vi "Automate_de_production.vi"(1 "OK Button 2":bool, 2 "Cancel Button 2":bool, 3 "?":bool, 4 "Cancel Button":bool, 5 "OK Button":bool, 6 "Radio Buttons":enum32{"Radio Selection 1", "Radio Selection 2"}(radio), 7 "StartB":bool) -> (0 "cannettes produites":dbl)   [LabVIEW 2023]
uses:
  Control 1.ctl
  Control 5.ctl
  <vilib>/numeric/Random Number (Range) U64.vi
  <vilib>/numeric/sub_Random U32.vi
panel:
  out "Produits defectueux":dbl
  out "Produits Finis":dbl
  out "Nb cycles":dbl
  in  "OK Button 3":bool
  out "MP3 2":bool
  out "Valeur PH":dbl
  out "Boolean":bool
  in  "Seuil PH":dbl(slide) scale=0.0..14.0
  out "Tab Control":T1(tab)
  out "MP3":bool
  out "Tank":cluster{dbl, dbl}(slide)={0.0, 10.0} scale=0.0..10.0
  # "DO u want gaz ?"
  # "DO u want sugar ?"
  # "Production finie"
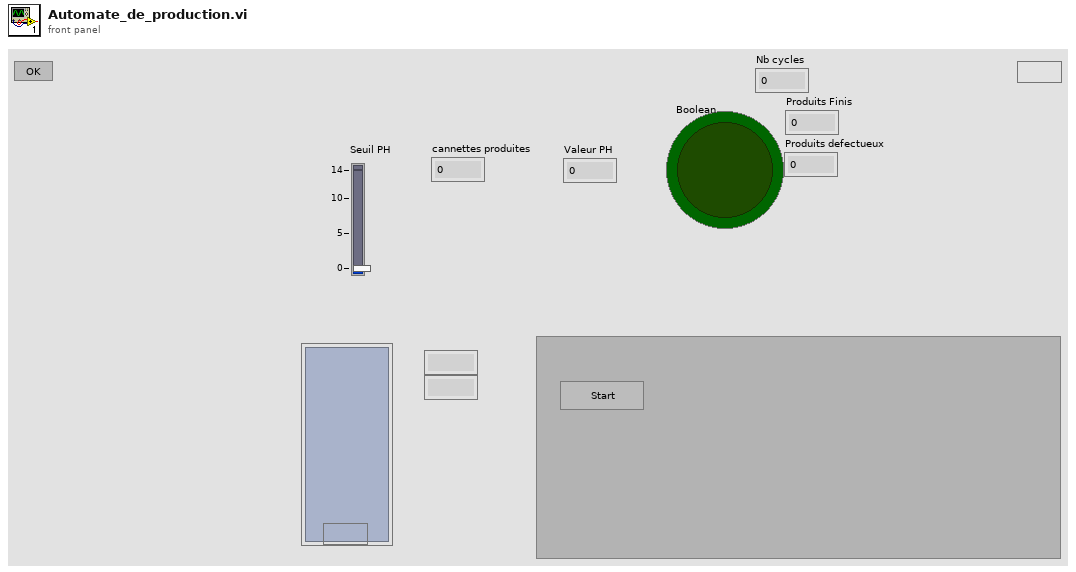
[diagram p1: front panel]
types:
  T1 = enum32{"Start", "Type", "preparer", "GazS", "GazF", "Sugar", "Finish"}
  T2 = typedef "Control 1.ctl" = enum32{"Start", "Page 1", "Page 2", "Page 3", "Page 4", "Sugar", "Finish"}
  T3 = typedef "Control 5.ctl" = enum32{"Start", "Page 1", "Page 2", "Page 3", "Page4"}
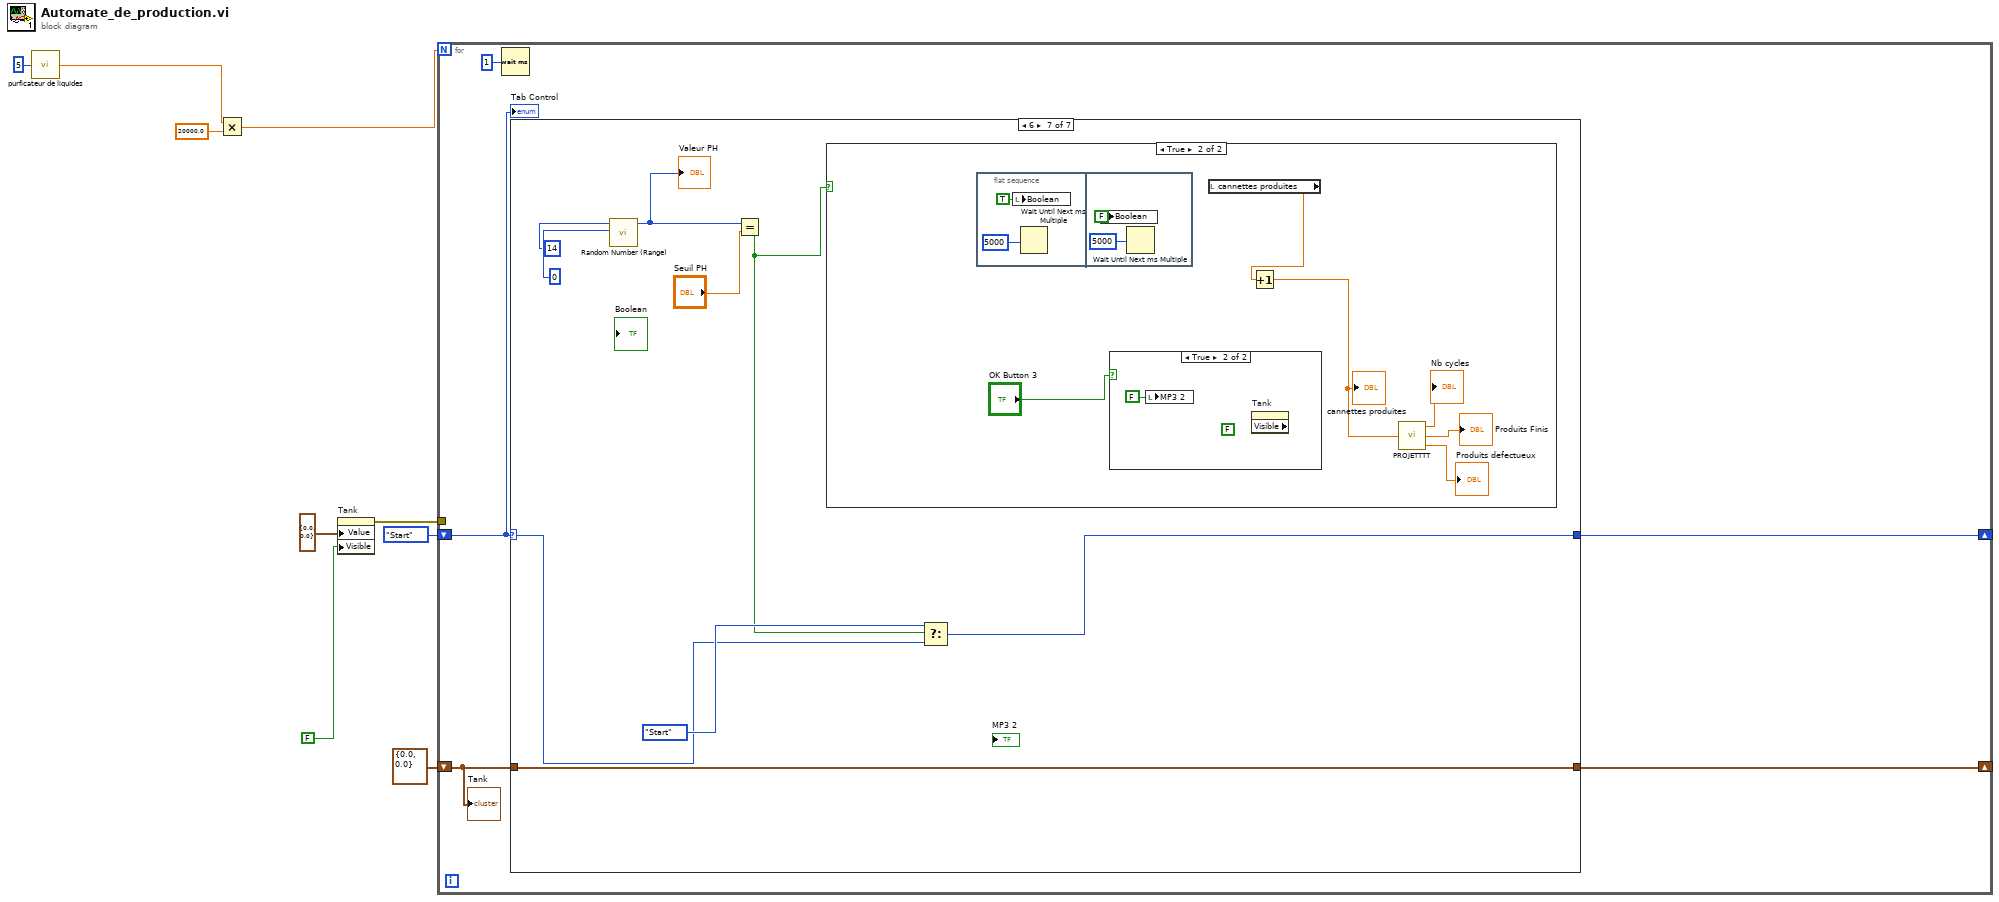
[diagram p0: block diagram]
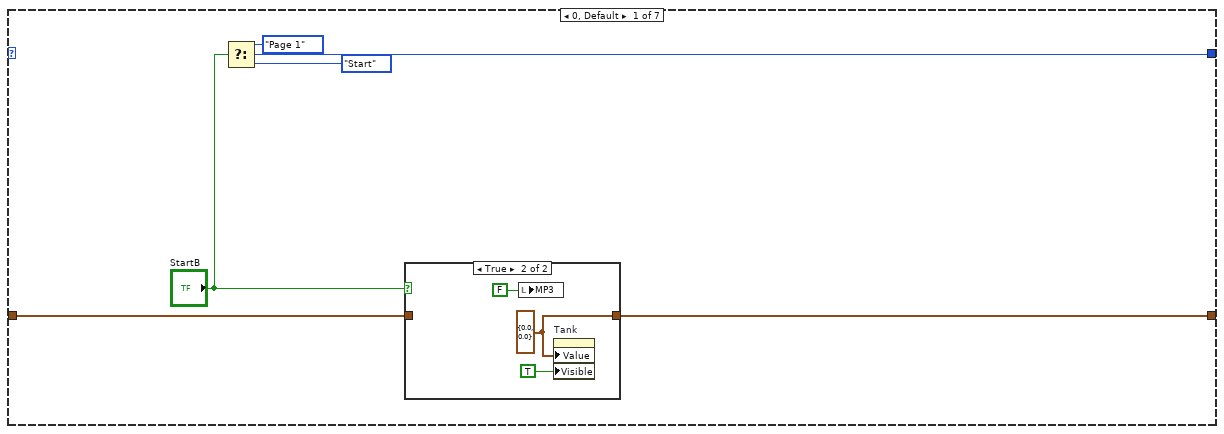
[diagram p2: hidden frame]
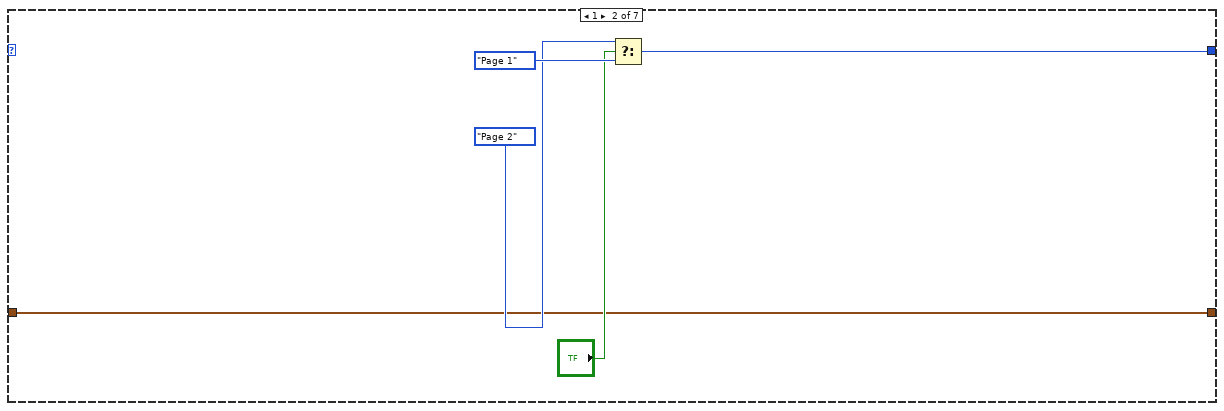
[diagram p4: hidden frame]
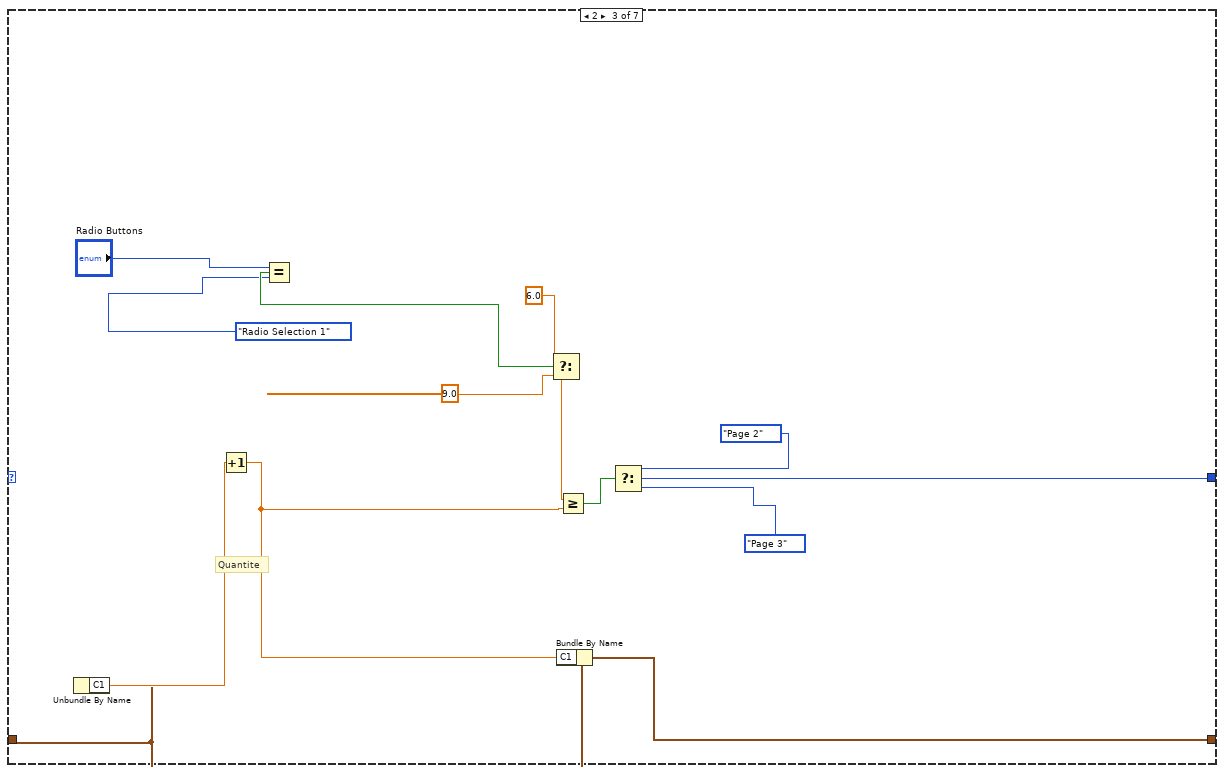
[diagram p5: hidden frame]
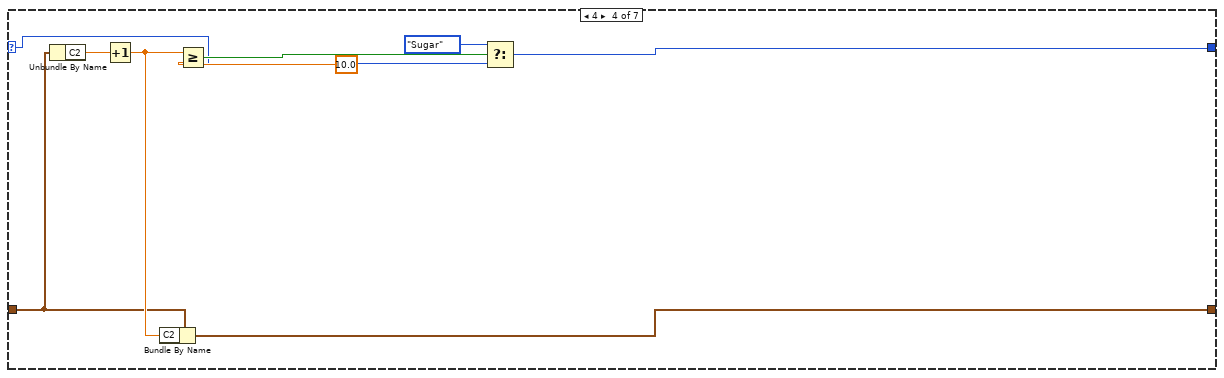
[diagram p6: hidden frame]
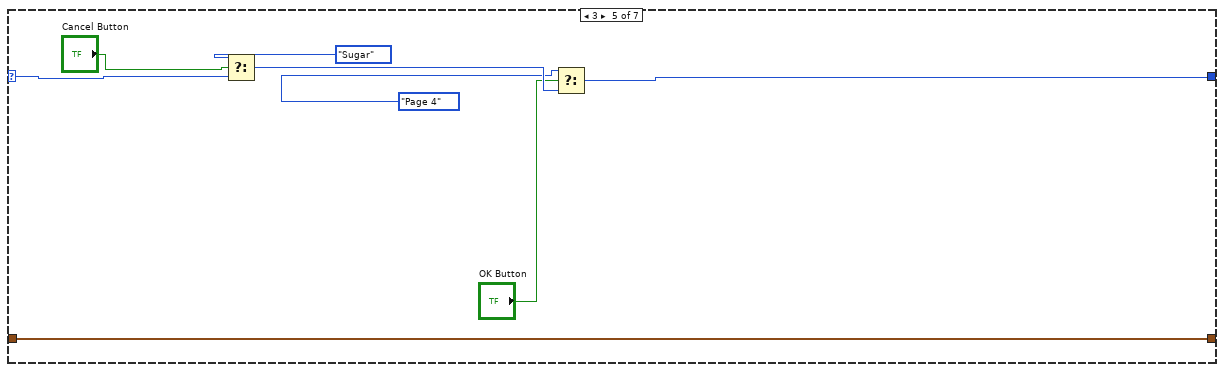
[diagram p7: hidden frame]
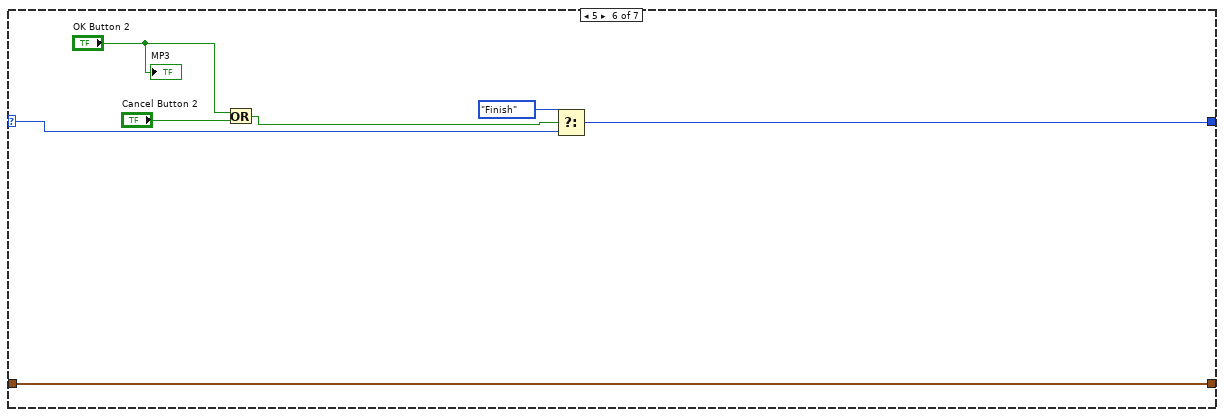
[diagram p8: hidden frame]
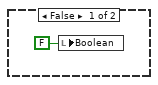
[diagram p9: hidden frame]
diagram:
  n1 = call "purficateur de liquides.vi"("Nb de litres recus"=5) -> ("nb de litres purifies"=w2:dbl)
  n2 = Multiply(x=w2, y=20000.0) -> (x*y=w3:dbl)
  n3 = property on="Tank" class="Slide (strict)"("Value"=cluster{dbl, dbl} {0.0, 0.0} ("Tank"), "Visible"=FALSE) -> (error out=w6:errorcluster)  [unwired: 2 in, 1 out]
  n4 = for {
    N: w3 -> [_]
    shift-right: [w14] -> _
    shift-left: cluster{"C1":dbl, "C2":dbl} {"C1"=0.0, "C2"=0.0} ("Tank") -> [w11]
    shift-right: [w12] -> _
    shift-left: Control_1."Start" ("Tab Control") -> [w13]
    tunnel: w6 -> [_]
    n5 = Wait (ms)(milliseconds to wait=u32 1 ("millisecond timer value")) -> ()  [unwired: 1 out]
    n6 = case shown="6" w13 {
      selector: w13 -> [_ _ _ w46 w59 w65 w74]
      tunnel: [w17 w26 w32 w44 w56 w62 w73] -> w12
      tunnel: w11 -> [w16 w25 w37 w48 w53 w67 w76]
      tunnel: [w15 w25 w36 w47 w53 w67 w76] -> w14
      frame 0, Default {
        n7 = Select(t=Control_5."Page 1" ("Tab Control"), s="StartB", f=Control_5."Start" ("Tab Control")) -> (s? t:f=w17:T3)
        n8 = case shown="True" "StartB" {
          tunnel: [w21 w22] -> w15
          tunnel: w16 -> [w21 _]
          frame False {
          }
          frame True {
            w22 = cluster{dbl, dbl} {0.0, 0.0} ("Tank")
            n9 = local write "MP3"(FALSE ("MP3")) -> ()
            n10 = property on="Tank" class="Slide (strict)"("Value"=w22, "Visible"=TRUE) -> ()  [unwired: 2 in, 2 out]
          }
        }
      }
      frame 1 {
        n11 = Select(t=Control_5."Page 2" ("Tab Control"), s="?", f=Control_5."Page 1" ("Tab Control")) -> (s? t:f=w26:T3)
      }
      frame 2 {
        # "Quantite"
        n12 = Unbundle By Name(w37) -> ("C1"=w38:dbl)
        n13 = Increment(x=w38) -> (x+1=w31:dbl)
        n14 = Equal?(x="Radio Buttons", y=enum32{"Radio Selection 1", "Radio Selection 2"}."Radio Selection 1" ("x")) -> (x = y?=w41:bool)
        n15 = Select(t=6.0, s=w41, f=9.0) -> (s? t:f=w30:dbl)
        n16 = Bundle By Name(cluster=w37, "C1"=w31) -> (w36:cluster{"C1":dbl, "C2":dbl})
        n17 = Greater Or Equal?(x=w30, y=w31) -> (x >= y?=w33:bool)
        n18 = Select(t=Control_5."Page 2" ("Tab Control"), s=w33, f=Control_5."Page 3" ("Tab Control")) -> (s? t:f=w32:T3)
      }
      frame 4 {
        n19 = Unbundle By Name(w48) -> ("C2"=w52:dbl)
        n20 = Increment(x=w52) -> (x+1=w51:dbl)
        n21 = Bundle By Name(cluster=w48, "C2"=w51) -> (w47:cluster{"C1":dbl, "C2":dbl})
        n22 = Greater Or Equal?(x=w51, y=10.0) -> (x >= y?=w50:bool)
        n23 = Select(t=Control_1."Sugar" ("Tab Control"), s=w50, f=w46) -> (s? t:f=w44:u32)
      }
      frame 3 {
        n24 = Select(t=Control_1."Sugar" ("Tab Control"), s="Cancel Button", f=w59) -> (s? t:f=w58:u32)
        n25 = Select(t=Control_1."Page 4" ("Tab Control"), s="OK Button", f=w58) -> (s? t:f=w56:u32)
      }
      frame 5 {
        n26 = Or(x="OK Button 2", y="Cancel Button 2") -> (x .or. y?=w64:bool)
        n27 = Select(t=Control_1."Finish" ("Tab Control"), s=w64, f=w65) -> (s? t:f=w62:u32)
        "MP3" <- "OK Button 2"
      }
      frame 6 {
        n28 = call-poly <vilib>:"Random Number (Range).vi"("lower bound (0)"=u64 0, "upper bound (100)"=u64 14) -> ("number"=w72:u64)  [unwired: 9 in]
        "Valeur PH" <- w72
        n29 = Equal?(x=w72, y="Seuil PH") -> (x = y?=w68:bool)
        n30 = case shown="True" w68 {
          frame False {
            n31 = local write "Boolean"(FALSE ("Boolean")) -> ()
          }
          frame True {
            n32 = flat-sequence {
              frame #0 {
                n33 = local write "Boolean"(TRUE ("Boolean")) -> ()
                n34 = Wait Until Next ms Multiple(millisecond multiple=u32 5000 ("millisecond timer value")) -> ()  [unwired: 1 out]
              }
              frame #1 {
                n35 = local write "Boolean"(FALSE ("Boolean")) -> ()
                n36 = Wait Until Next ms Multiple(millisecond multiple=u32 5000 ("millisecond timer value")) -> ()  [unwired: 1 out]
              }
            }
            n37 = case shown="True" "OK Button 3" {
              frame False {
              }
              frame True {
                (unwired) FALSE ("Visible")
                n38 = local write "MP3 2"(FALSE ("MP3")) -> ()
                n39 = property on="Tank" class="Slide (strict)" props=["Visible"]() -> ()  [unwired: 2 in, 3 out]
              }
            }
            n40 = local read "cannettes produites"() -> (w83:dbl)
            n41 = Increment(x=w83) -> (x+1=w81:dbl)
            "cannettes produites" <- w81
            n42 = call "PROJETTTT.vi"("Numérique"=w81) -> ("Nb cycles"=→"Nb cycles":dbl, "Produits Finis"=→"Produits Finis":dbl, "Produits defectueux"=→"Produits defectueux":dbl)
          }
        }
        n43 = Select(t=Control_1."Start" ("Tab Control"), s=w68, f=w74) -> (s? t:f=w73:u32)
      }
    }
    "Tab Control" <- w13
    "Tank" <- w11
  }
